vi "ElcomXP.vi"(3 "Input":string[](array[string])) -> (0 "output variable":dbl, 1 "Elcom XP":dbl, 2 "Slide":i8(slide) scale=0.0..15.0)   [LabVIEW 2014]
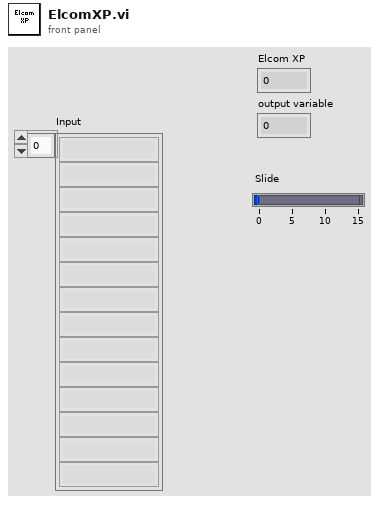
[diagram p1: front panel]
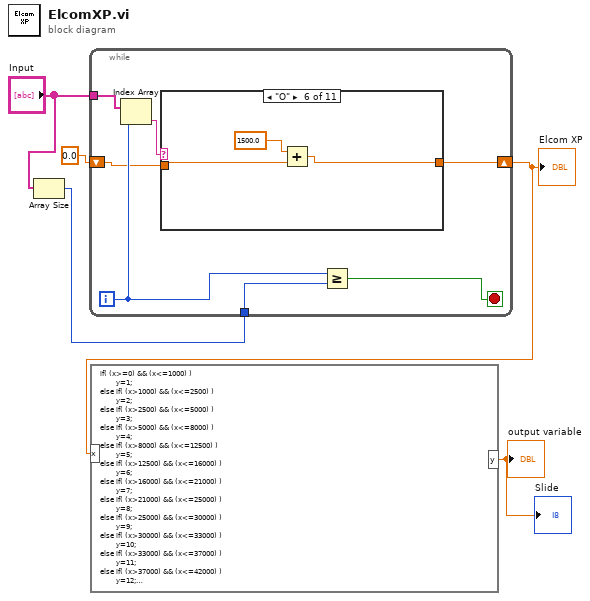
[diagram p0: block diagram]
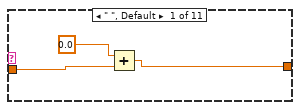
[diagram p2: hidden frame]
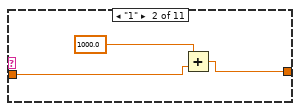
[diagram p3: hidden frame]
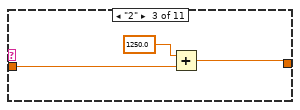
[diagram p4: hidden frame]
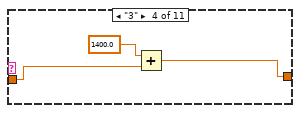
[diagram p5: hidden frame]
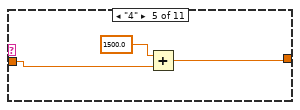
[diagram p6: hidden frame]
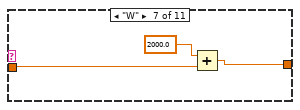
[diagram p7: hidden frame]
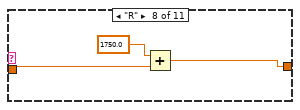
[diagram p8: hidden frame]
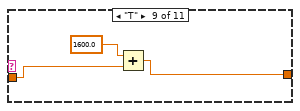
[diagram p9: hidden frame]
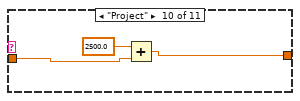
[diagram p10: hidden frame]
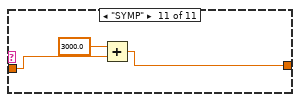
[diagram p11: hidden frame]
diagram:
  n1 = Array Size(array="Input") -> (size(s)=w3:i32)
  n2 = while {
    tunnel: "Input" -> [w10]
    tunnel: w3 -> [w12]
    shift-right: [w6] -> w2
    shift-left: 0.0 ("Numeric") -> [w7]
    i -> [w9]
    stop <- w11 stop-if-true
    n3 = Index Array(array=w10, index=w9) -> (element=w8:string)
    n4 = case shown="\"O\"" w8 {
      tunnel: w7 -> [w14 w17 w20 w23 w26 w29 w32 w35 w38 w41 w45]
      tunnel: [w13 w16 w19 w22 w25 w28 w31 w34 w37 w40 w43] -> w6
      frame " ", Default {
        n5 = Add(x=0.0 ("Numeric"), y=w14) -> (x+y=w13:dbl)
      }
      frame "1" {
        n6 = Add(x=1000.0 ("Numeric"), y=w17) -> (x+y=w16:dbl)
      }
      frame "2" {
        n7 = Add(x=1250.0 ("Numeric"), y=w20) -> (x+y=w19:dbl)
      }
      frame "3" {
        n8 = Add(x=1400.0 ("Numeric"), y=w23) -> (x+y=w22:dbl)
      }
      frame "4" {
        n9 = Add(x=1500.0 ("Numeric"), y=w26) -> (x+y=w25:dbl)
      }
      frame "O" {
        n10 = Add(x=1500.0 ("Numeric"), y=w29) -> (x+y=w28:dbl)
      }
      frame "W" {
        n11 = Add(x=2000.0 ("Numeric"), y=w32) -> (x+y=w31:dbl)
      }
      frame "R" {
        n12 = Add(x=1750.0 ("Numeric"), y=w35) -> (x+y=w34:dbl)
      }
      frame "T" {
        n13 = Add(x=1600.0 ("Numeric"), y=w38) -> (x+y=w37:dbl)
      }
      frame "Project" {
        n14 = Add(x=2500.0, y=w41) -> (x+y=w40:dbl)
      }
      frame "SYMP" {
        n15 = Add(x=3000.0, y=w45) -> (x+y=w43:dbl)
      }
    }
    n16 = Greater Or Equal?(x=w9, y=w12) -> (x >= y?=w11:bool)
  }
  "Elcom XP" <- w2
  n17 = formula code="if( (x>=0) && (x<=1000) )\n        y=1;\nelse if( (x>1000) && (x<=2500) )\n        y=2;\nelse if( (x>2500) && (x<=5000) )\n        y=3;\nelse if( (x>5000) && (x<=8000) )\n        y=4;\nelse if( (x>8000) && (x<=12500) )\n        y=5;\nelse if( (x>12500) && (x<=16000) )\n        y=6;\nelse if( (x>16000) && (x<=21000) )\n        y=7;\nelse if( (x>21000) && (x<=25000) )\n        y=8;\nelse if( (x>25000) && (x<=30000) )\n        y=9;\nelse if( (x>30000) && (x<=33000) )\n        y=10;\nelse if( (x>33000) && (x<=37000) )\n        y=11;\nelse if( (x>37000) && (x<=42000) )\n        y=12;\nelse if( (x>42000) && (x<=45000) )\n        y=13;\nelse if( (x>45000) && (x<=47500) )\n        y=14;\nelse if( (x>47500) && (x<=50000) )\n        y=15;"("x"=w2) -> ("y"=→"output variable" →"Slide":dbl)
